vi "Get Pulse State.vi"(8 "error in (no error)":errorcluster, 11 "NI-Scope Digitizer in":refnum<class "Ni-Scope Digitizer.lvclass">) -> (0 "error out":errorcluster, 1 "Data ready":bool, 2 "Armed":bool, 3 "NI-Scope Digitizer out":refnum<class "Ni-Scope Digitizer.lvclass">, 4 "Recording compleste":bool)   [LabVIEW 2021, in "Ni-Scope Digitizer.lvclass"]
uses:
  Ni-Scope Digitizer.lvclass
  Ni-Scope Digitizer.lvclass/Ni-Scope Digitizer.ctl
panel:
  out "Availiable Samples":u32
  out "Finished":bool
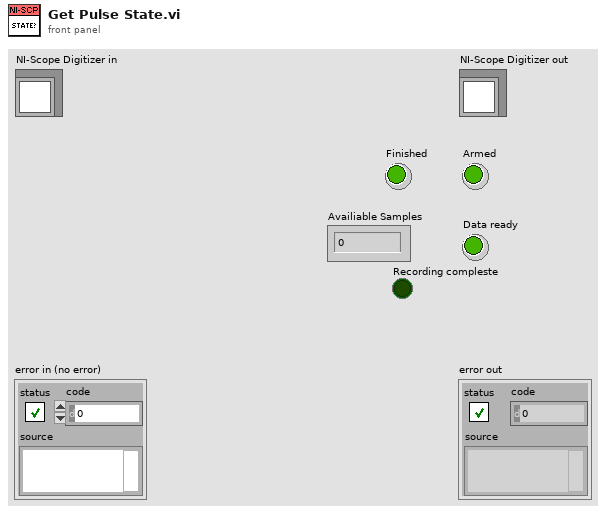
[diagram p1: front panel]
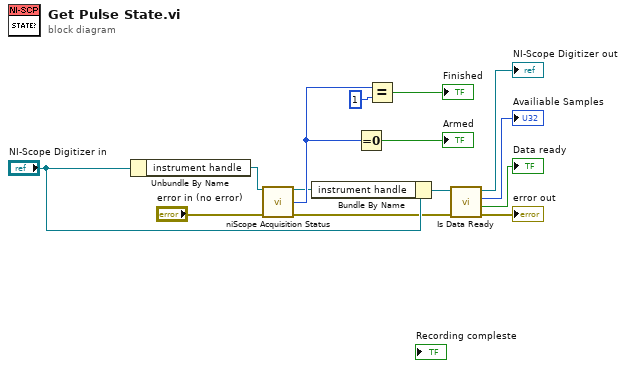
[diagram p0: block diagram]
diagram:
  n1 = Unbundle By Name("NI-Scope Digitizer in") -> ("instrument handle"=w14:refnum<k15>)
  n2 = call <instrlib>:"niScope Acquisition Status.vi"("instrument handle"=w14, "error in"="error in (no error)") -> ("instrument handle out"=w7:refnum<k15>, "acquisition status"=w11:i32, "error out"=w2:errorcluster)  [unwired: 11 out]
  n3 = Bundle By Name(cluster="NI-Scope Digitizer in", "instrument handle"=w7) -> (w6:refnum<class "Ni-Scope Digitizer.lvclass">)
  n4 = Equal To 0?(x=w11) -> (x = 0?=→"Armed":bool)
  n5 = Equal?(x=w11, y=1) -> (x = y?=→"Finished":bool)
  n6 = call-dynamic "Is Data Ready.vi"("error in (no error)"=w2, "Ni-Scope Digitizer in"=w6) -> ("error out"=→"error out":errorcluster, "Data ready"=→"Data ready":bool, "Availiable Samples"=→"Availiable Samples":u32, "Ni-Scope Digitizer out"=→"NI-Scope Digitizer out":refnum<class "Ni-Scope Digitizer.lvclass">)  [unwired: 6 in]
